vi "DD_RunScript_TS_Step.vi"(0 "Engine Reference":refnum<k7>, 1 "Script Path":string, 2 "Precondition":string, 5 "Sequence File Ref":refnum<k7>, 7 "Step Name":string="Run Script", 9 "Requirement":string, 11 "error in":errorcluster, 12 "index":i32) -> (4 "Engine reference(out)":refnum<k7>, 6 "Sequence File Ref(out)":refnum<k7>, 15 "error out":errorcluster)   [LabVIEW 2010]
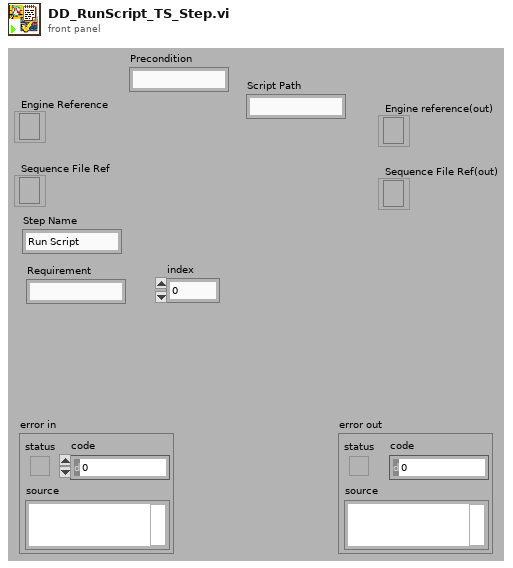
[diagram p1: front panel]
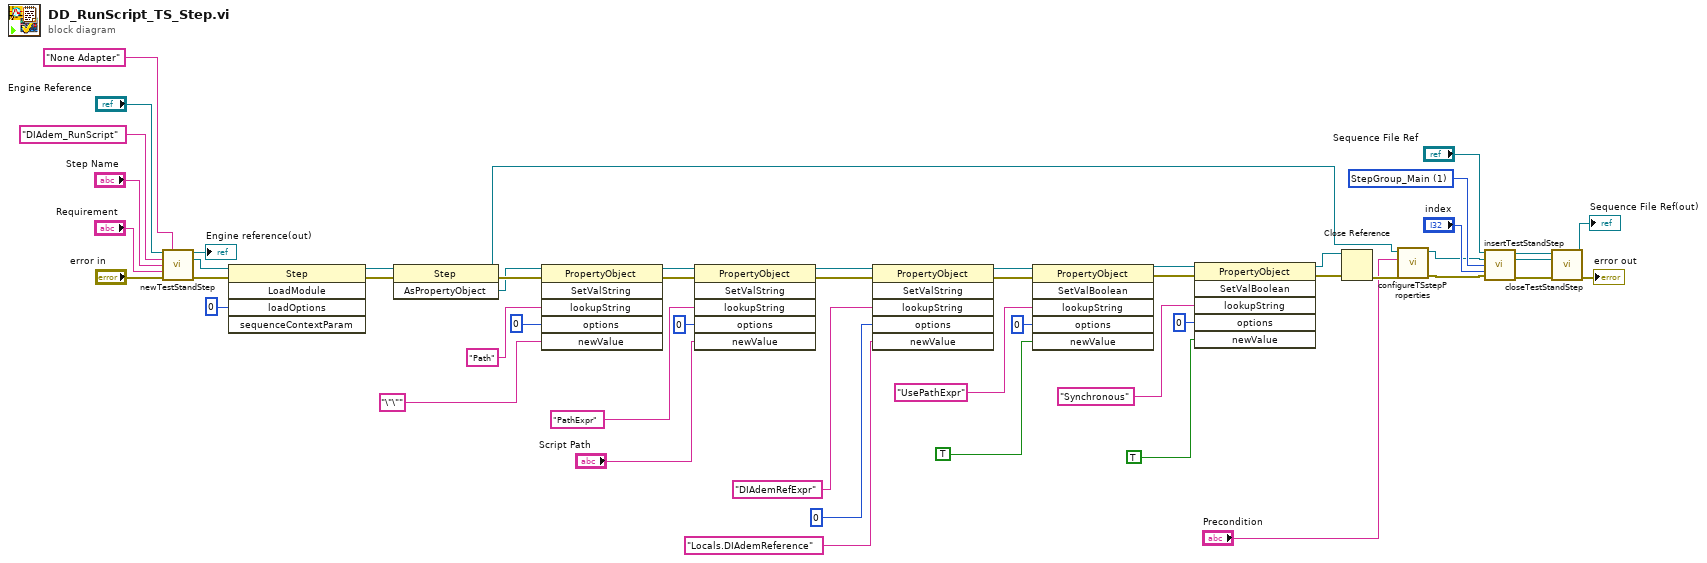
[diagram p0: block diagram]
diagram:
  w38 = 1 items=["StepGroup_Setup", "StepGroup_Main", "StepGroup_Cleanup"] ("Step Group")
  n1 = call "newTestStandStep.vi"("Engine reference"="Engine Reference", "adapterKeyNameVal"="None Adapter", "stepType"="DIAdem_RunScript", "Step Name"="Step Name", "Requirement"="Requirement", "error in"="error in") -> ("Engine reference(out)"=→"Engine reference(out)":refnum<k7>, "NewStep (out)"=w35:refnum<k7>, "error out"=w36:errorcluster)  [unwired: 7 in]
  n2 = invoke class="Step" method="LoadModule"(reference=w35, error in=w36, "loadOptions"=0) -> (reference out=w43:refnum<k7>, error out=w44:errorcluster)  [unwired: 2 in, 3 out]
  n3 = invoke class="Step" method="AsPropertyObject"(reference=w43, error in=w44) -> (reference out=w3:refnum<k7>, error out=w46:errorcluster, "AsPropertyObject"=w45:refnum<k7>)  [unwired: 1 in]
  n4 = invoke class="PropertyObject" method="SetValString"(reference=w45, error in=w46, "lookupString"="Path", "options"=0, "newValue"="\"\"" ("Source Data")) -> (reference out=w27:refnum<k7>, error out=w26:errorcluster)  [unwired: 1 in, 4 out]
  n5 = invoke class="PropertyObject" method="SetValString"(reference=w27, error in=w26, "lookupString"="PathExpr", "options"=0, "newValue"="Script Path") -> (reference out=w22:refnum<k7>, error out=w21:errorcluster)  [unwired: 1 in, 4 out]
  n6 = invoke class="PropertyObject" method="SetValString"(reference=w22, error in=w21, "lookupString"="DIAdemRefExpr", "options"=0, "newValue"="Locals.DIAdemReference") -> (reference out=w20:refnum<k7>, error out=w19:errorcluster)  [unwired: 1 in, 4 out]
  n7 = invoke class="PropertyObject" method="SetValBoolean"(reference=w20, error in=w19, "lookupString"="UsePathExpr", "options"=0, "newValue"=TRUE ("Use Name?")) -> (reference out=w13:refnum<k7>, error out=w12:errorcluster)  [unwired: 1 in, 4 out]
  n8 = invoke class="PropertyObject" method="SetValBoolean"(reference=w13, error in=w12, "lookupString"="Synchronous", "options"=0, "newValue"=TRUE ("CreateChannel?")) -> (reference out=w14:refnum<k7>, error out=w15:errorcluster)  [unwired: 1 in, 4 out]
  n9 = Close Reference(reference=w14, error in (no error)=w15) -> (error out=w5:errorcluster)
  n10 = call "configureTSstepProperties.vi"("error in"=w5, "Precondition"="Precondition", "NewStep (in)"=w3) -> ("error out"=w4:errorcluster, "NewStep (out)"=w2:refnum<k7>)  [unwired: 7 in]
  n11 = call "insertTestStandStep.vi"("Sequence File Ref"="Sequence File Ref", "Step to insert"=w2, "Step Group"=w38, "index"="index", "error out"=w4) -> ("Sequence File Ref(out)"=w8:refnum<k7>, "Step to insert (out)"=w7:refnum<k7>, "error out"=w40:errorcluster)  [unwired: 8 in]
  n12 = call "closeTestStandStep.vi"("error in"=w40, "NewStep"=w7, "Sequence File Ref"=w8) -> ("error out"=→"error out":errorcluster, "Sequence File Ref(out)"=→"Sequence File Ref(out)":refnum<k7>)  [unwired: 7 in]
